vi "Write.vi"(0 "session in":T1[](array[typedef]) {"rx baseband session"."3630 session"."Address Space" items=["VXI/VME A16"=1, "VXI/VME A24"=2, "VXI/VME A32"=3, "VXI/VME A64"=4, "PXI Memory Allocations"=9, "PXI Configuration"=10, "PXI BAR0"=11, "PXI BAR1"=12, "PXI BAR2"=13, "PXI BAR3"=14, "PXI BAR4"=15, "PXI BAR5"=16]; "tx baseband session"."3610 session"."Address Space" items=["VXI/VME A16"=1, "VXI/VME A24"=2, "VXI/VME A32"=3, "VXI/VME A64"=4, "PXI Memory Allocations"=9, "PXI Configuration"=10, "PXI BAR0"=11, "PXI BAR1"=12, "PXI BAR2"=13, "PXI BAR3"=14, "PXI BAR4"=15, "PXI BAR5"=16]}, 1 "memo":enum16{"DRAM", "BRAM"}(ring), 5 "data":i16[](array[numeric]), 7 "Wfm addr":u32, 9 "zero pad":bool, 11 "error in":errorcluster) -> (3 "burst memo":enum16{"DRAM", "BRAM"}(ring), 4 "session out":T1[](array[typedef]) {"rx baseband session"."3630 session"."Address Space" items=["VXI/VME A16"=1, "VXI/VME A24"=2, "VXI/VME A32"=3, "VXI/VME A64"=4, "PXI Memory Allocations"=9, "PXI Configuration"=10, "PXI BAR0"=11, "PXI BAR1"=12, "PXI BAR2"=13, "PXI BAR3"=14, "PXI BAR4"=15, "PXI BAR5"=16]; "tx baseband session"."3610 session"."Address Space" items=["VXI/VME A16"=1, "VXI/VME A24"=2, "VXI/VME A32"=3, "VXI/VME A64"=4, "PXI Memory Allocations"=9, "PXI Configuration"=10, "PXI BAR0"=11, "PXI BAR1"=12, "PXI BAR2"=13, "PXI BAR3"=14, "PXI BAR4"=15, "PXI BAR5"=16]}, 6 "last wr addr":u32, 15 "error out":errorcluster)   [LabVIEW 2019, in "mmWave HW Control.lvlib"]
uses:
  mmWave HW Control.lvlib
  Low-level/TypeDefs/Session.ctl
  <instrlib>/niMmWave/ni3620/Config/v1/Host/Public/High-Level/niMmWave Session.ctl
  <instrlib>/_niInstr/Register Bus/v0/Host/Public/Register Bus Session.ctl
  <instrlib>/_niInstr/Register Bus/v0/Host/Private/Session Data.ctl
  <instrlib>/niMmWave/ni3620/Config/v1/Host/Public/Typedefs/Board Information.ctl
  <instrlib>/niMmWave/ni3620/Config/v1/Host/Public/Typedefs/Hardware Revision.ctl
  <instrlib>/niMmWave/ni3620/Config/v1/Host/Public/Typedefs/Gain Mapping.ctl
  <instrlib>/niMmWave/ni3620/Config/v1/Host/Public/Typedefs/Correction Data.ctl
  <instrlib>/niMmWave/ni3620/Config/v1/Host/Public/Typedefs/Opera Characterization.ctl
  <instrlib>/niMmWave/ni3620/Config/v1/Host/Public/Corrections/Typedefs/Opera Characterization Main Header.ctl
  <instrlib>/niMmWave/ni3620/Config/v1/Host/Public/Corrections/Typedefs/Opera IF Board Information.ctl
  <instrlib>/niMmWave/ni3620/Config/v1/Host/Public/Corrections/Typedefs/Opera Characterization Instance Header.ctl
  <instrlib>/niMmWave/ni3620/Config/v1/Host/Public/Corrections/Typedefs/Opera Characterization Device Data Header.ctl
  <instrlib>/niMmWave/ni3620/Config/v1/Host/Public/Corrections/Typedefs/Opera LO Characterization Data Header.ctl
  <instrlib>/niMmWave/ni3620/Config/v1/Host/Public/Corrections/Typedefs/Opera IF Board Characterization Data Header.ctl
  <instrlib>/niMmWave/ni3620/Config/v1/Host/Public/Corrections/Typedefs/Opera Characterization Device Data.ctl
  <instrlib>/niMmWave/ni3620/Config/v1/Host/Public/Corrections/Typedefs/Opera LO2 Board Characterization Data.ctl
  <instrlib>/niMmWave/ni3620/Config/v1/Host/Public/Corrections/Typedefs/Opera LO Characterization Data.ctl
  <instrlib>/niMmWave/ni3620/Config/v1/Host/Public/Corrections/Typedefs/Opera IF Board Characterization Data.ctl
  <instrlib>/niMmWave/ni3620/Config/v1/Host/Public/Corrections/Typedefs/Opera IQ Impairment Data.ctl
  <instrlib>/niMmWave/ni3620/Config/v1/Host/Public/Typedefs/mmWave Adapter Session Data.ctl
  <instrlib>/niMmWave/ni3620/Config/v1/Host/Public/Typedefs/mmWave Adapter Data.ctl
  <instrlib>/niMmWave/ni3620/Config/v1/Host/Public/Typedefs/mmWave Adapter 2.ctl
  <instrlib>/niMmWave/ni3620/Config/v1/Shared/Typedefs/Subsystem ID.ctl
  <instrlib>/niMmWave/ni3620/Config/v1/Host/Public/Typedefs/mmWave Adapter Channel Information.ctl
  <instrlib>/niMmWave/ni3620/Config/v1/Host/Public/Typedefs/Temperature Coefficients.ctl
  <instrlib>/niMmWave/ni3620/Config/v1/Host/Public/Typedefs/mmWave Characterization.ctl
  <instrlib>/niMmWave/ni3620/Config/v1/Host/Public/Corrections/Typedefs/mmWave Characterization Main Header.ctl
  <instrlib>/niMmWave/ni3620/Config/v1/Host/Public/Corrections/Typedefs/mmWave Characterization Instance Header.ctl
  <instrlib>/niMmWave/ni3620/Config/v1/Host/Public/Typedefs/Session Cache.ctl
  <instrlib>/niMmWave/ni3620/Config/v1/Host/Public/Typedefs/LO2 settings cache.ctl
  <instrlib>/niMmWave/ni3620/Config/v1/Host/Public/Typedefs/LO2 source.ctl
  <instrlib>/niMmWave/ni3620/Config/v1/Host/Public/Typedefs/Desired and Coerced.ctl
  <instrlib>/niMmWave/ni3620/Config/v1/Host/Public/Typedefs/Export cache.ctl
  <instrlib>/niMmWave/ni3620/Config/v1/Host/Public/Typedefs/Path cache.ctl
  <instrlib>/niMmWave/ni3620/Config/v1/Host/Public/Typedefs/Daughterboard Type.ctl
  <instrlib>/niMmWave/ni3620/Config/v1/Host/Public/Typedefs/LO1 settings cache.ctl
  <instrlib>/niMmWave/ni3620/Config/v1/Host/Public/Typedefs/LO1 Source.ctl
  <instrlib>/niMmWave/ni3620/Config/v1/Host/Public/Typedefs/mmWave export cache.ctl
  <instrlib>/niMmWave/ni3620/Config/v1/Host/Private/Board/LO2/LO2 Board Configuration Cache.ctl
  <instrlib>/niMmWave/ni3620/Config/v1/Host/Public/Typedefs/reference clock routing settings.ctl
  <instrlib>/niMmWave/ni3620/Config/v1/Host/Public/Typedefs/LO2 routing settings.ctl
  <instrlib>/niMmWave/ni3620/Config/v1/Host/Private/Board/LO1/LO1 Board Configuration Cache.ctl
  <instrlib>/niMmWave/ni3620/Config/v1/Host/Public/Typedefs/LO1 source settings.ctl
  <instrlib>/niMmWave/ni3620/Config/v1/Host/Public/Typedefs/LO1 export settings.ctl
  <instrlib>/niMmWave/ni3620/Config/v1/Host/Public/Typedefs/LO1 mmWave settings.ctl
  Low-level/TypeDefs/Tx Baseband Session.ctl
  <instrlib>/niMmWave/ni3610 and ni3630/controls/public/Main Settings.ctl
  <vilib>/Instr/_visa.llb/VISA Register Access Address Space.ctl
  <instrlib>/niMmWave/ni3610 and ni3630/controls/public/Register Adresses.ctl
  <instrlib>/niMmWave/ni3610 and ni3630/controls/public/Base Card Type.ctl
  <instrlib>/niMmWave/ni3610 and ni3630/controls/private/IQ Card Revision.ctl
  <instrlib>/niMmWave/ni3610 and ni3630/controls/public/Board Capability.ctl
  Low-level/TypeDefs/Blank FPGA Reference.ctl
  Low-level/TypeDefs/Rx Baseband Session.ctl
  Low-level/TypeDefs/Hardware Configuration.ctl
  Low-level/TypeDefs/Direction.ctl
  Low-level/TypeDefs/Gain Ranging.ctl
  Low-level/TypeDefs/PXI Trigger Bus Info.ctl
  Low-level/TypeDefs/TX driver FPGA ref.ctl
  00e56df4-ad1d-4d91-93ea-fba1cea4a9f5.vi
  38a8d631-9b78-4ee6-a370-a9c59af1ef2c.vi
  705eeaa0-497a-4033-9a85-e633e8683a5e.vi
  0942d1b7-6fcb-43fb-bb48-4a735e411df6.vi
  <vilib>/Utility/High Resolution Relative Seconds.vi
  <vilib>/Utility/error.llb/Clear Errors.vi
  <vilib>/rvi/errors/niLvFpgaAdjustHostInterfaceError.vi
  <vilib>/rvi/interface/common/niFpgaWaitOnOcc.vi
  <vilib>/rvi/interface/nirviReadWriteControl/nirviReadWriteControl.xnode
  <vilib>/rvi/interface/nirviMethod/nirviMethod.xnode
  NiFpgaLv.dll
  <vilib>/rvi/interface/Simulation/niFpgaSimulationCallBeginRW.vi
  <vilib>/rvi/errors/niLvFpgaMergeErrorWithErrorCode.vi
  <vilib>/FPGAPlugInAG/Dynamic/niLvFpga_ConfigureFifo_Dynamic.vi
  <vilib>/FPGAPlugInAG/Dynamic/niLvFpga_StartFifo_Dynamic.vi
  <vilib>/FPGAPlugInAG/Dynamic/niLvFpga_WriteFifo_Dynamic.vi
  <instrlib>/_niInstr/Register Bus/v0/Host/niInstr Register Bus v0 Host.lvlib
  <instrlib>/niMmWave/ni3610 and ni3630/ni3610_and_ni3630_Driver_Lib.lvlib
  <instrlib>/niMmWave/ni3620/Config/v1/Host/niMmWave Config v1 Host.lvlib
  <instrlib>/niMmWave/ni3620/Config/v1/Shared/niMmWave Config v1 Shared.lvlib
panel:
  out "conversion time":dbl format="%#_6p"
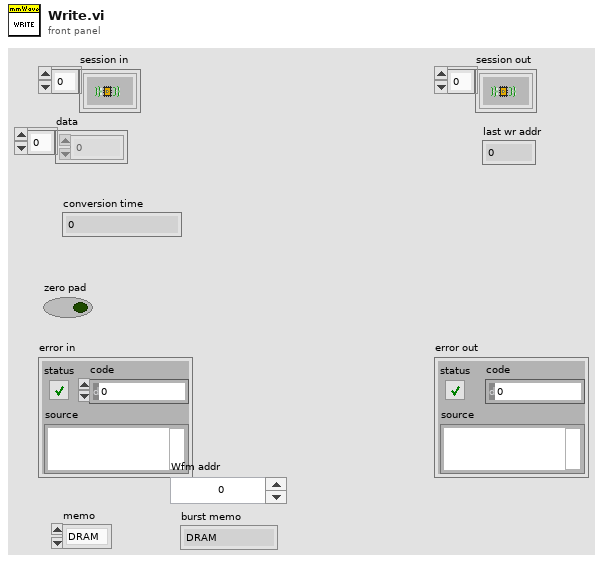
[diagram p1: front panel]
types:
  T1 = typedef "Session.ctl" = cluster{"3620 session":refnum<queue>, "tx baseband session":T2, "rx baseband session":T10, "tx gain (dB)":dbl, "rx gain (dB)":dbl, "hardware configuration":T11, "gain ranging":T13[], "pxi trigger bus information":T14}
  T2 = typedef "Tx Baseband Session.ctl" = cluster{"3610 session":T3, "7902 reference":T9}
  T3 = typedef "ni3610_and_ni3630_Driver_Lib.lvlib/Main Settings.ctl" = cluster{"VISA resource name":refnum<visa-resource-name>, "Address Space":T4, "window_offset":u32, "register_addresses":T5, "required_MM_fpga_version":cluster{"signature":u32, "hardware":u32, "current revision":u32, "oldest revision":u32}, "CPLD Oldest Compat Version ":cluster{"hardware":u32, "CPLD firmware":u32}, "MM_FPGA_image_location":string, "is_init":bool, "card_type":T6, "DacLmkConfigFileName":string, "AdcLmkConfigFileName":string, "AdcConfigFileName":string, "DacConfigFileName_RevA":string, "DacConfigFileName_RevB":string, "Mulde hardware revision":u8, "bypass DAC PLL\n":bool, "IQ Card Revision":T7, "board capability":T8}
  T4 = typedef "VISA Register Access Address Space.ctl" = u16
  T5 = typedef "ni3610_and_ni3630_Driver_Lib.lvlib/Register Adresses.ctl" = cluster{"MM based Registers":cluster{"Revision":u32, "OldestCompatRev":u32, "signature":u32, "scratch":u32, "LedControl":u32, "BoardHwRev":u32, "BoardControl":u32, "ThermalStatus":u32, "BasebandStatus":u32, "BasebandControl":u32, "BasebandAuxSetup":u32, "BasebandAuxStatus":u32, "LmkSyncOutSetup":u32, " AdcSyncOutSetup":u32, " InjSyncOutSetup":u32, " PxiTrig0OutSetup":u32, " PxiTrig1OutSetup":u32, " PxiTrig2OutSetup":u32, " PxiTrig3OutSetup":u32, " PxiTrig4OutSetup":u32, " PxiTrig5OutSetup":u32, " PxiTrig6OutSetup":u32, " PxiTrig7OutSetup":u32}, "CPLD based Registers":cluster{"SlaveSignature":u32, "SlaveRevision":u32, "SlaveOldestCompatRev":u32, "SlaveScratch":u32, "SlaveSetup":u32, "SlaveStatus":u32, "IDacReg_offset":u32, "LMKRegGrp0_offset":u32, "QDacReg_offset":u32, "BrdTempSensorVal":u32, "TempSensorPowerDown":u32, "GPIOReg_offset":u32, "IAdcReg_offset":u32, "QAdcReg_offset":u32, "LMKRegGrp1_offset":u32, "QadcTempSensorVal":u32, "IadcTempSensorVal":u32, "RevisionReg":u32, "VcxoReg":u32, "CpldStatusReg":u32, "PowerReg":u32, "VBiasEnReg":u32, "ExtRefOeReg":u32, "QdacCtrlReg":u32, "QdacStatusReg":u32, "IdacCtrlReg":u32, "IdacStatusReg":u32, "QdacJtagIn":u32, "QdacJtagOut":u32, "IdacJtagIn":u32, "IdacJtagOut":u32, "IqDcSetupReg":u32, "QadcStatusReg":u32, "IadcStatusReg":u32, "BrdSetupReg":u32, "IqDcRevisionReg":u32, "PllStatusReg":u32, "EndpointScratchReg":u32, "AdcSyncCfgReg":u32, "IqCardOpampReg":u32}, "CPLD Register Offset":u32, "MM  Register Offset":u32, " PxiTrig0OutSetup":u32}
  T6 = typedef "ni3610_and_ni3630_Driver_Lib.lvlib/Base Card Type.ctl" = enum16{"unspecified", "ADC", "DAC"}
  T7 = typedef "ni3610_and_ni3630_Driver_Lib.lvlib/IQ Card Revision.ctl" = enum16{"RevA", "RevB", "RevC", "RevD"}
  T8 = typedef "ni3610_and_ni3630_Driver_Lib.lvlib/Board Capability.ctl" = cluster{"baseband sync":enum16{"no baseband sync", "baseband sync"}}
  T9 = typedef "Blank FPGA Reference.ctl" = refnum<k20>
  T10 = typedef "Rx Baseband Session.ctl" = cluster{"3630 session":T3, "7902 reference":T9}
  T11 = typedef "Hardware Configuration.ctl" = cluster{"direction":T12, "baseband only":bool}
  T12 = typedef "Direction.ctl" = enum16{"Transceiver", "Receiver", "Transmitter"}
  T13 = typedef "Gain Ranging.ctl" = cluster{"gain ranging active scope":string, "gain ranging stream session":refnum<k20>}
  T14 = typedef "PXI Trigger Bus Info.ctl" = cluster{"chassis resource name":refnum<visa-resource-name>, "7902R (TX)":i16, "3610 (TX)":i16, "3620 (IF)":i16, "3630 (RX)":i16, "7902R (RX)":i16}
  T15 = cluster{"generation select":enum16{"Pass Through", "Tone", "Pulse", "Disable"}, "tone parameters":cluster{"frequency":fxp<+/-,48,0>, "gain":fxp<+/-,18,1>}, "pulse parameters":cluster{"frequency":u32, "gain":fxp<+/-,18,1>, "width":u8}}
  T16 = typedef "TX driver FPGA ref.ctl" = refnum<k20>
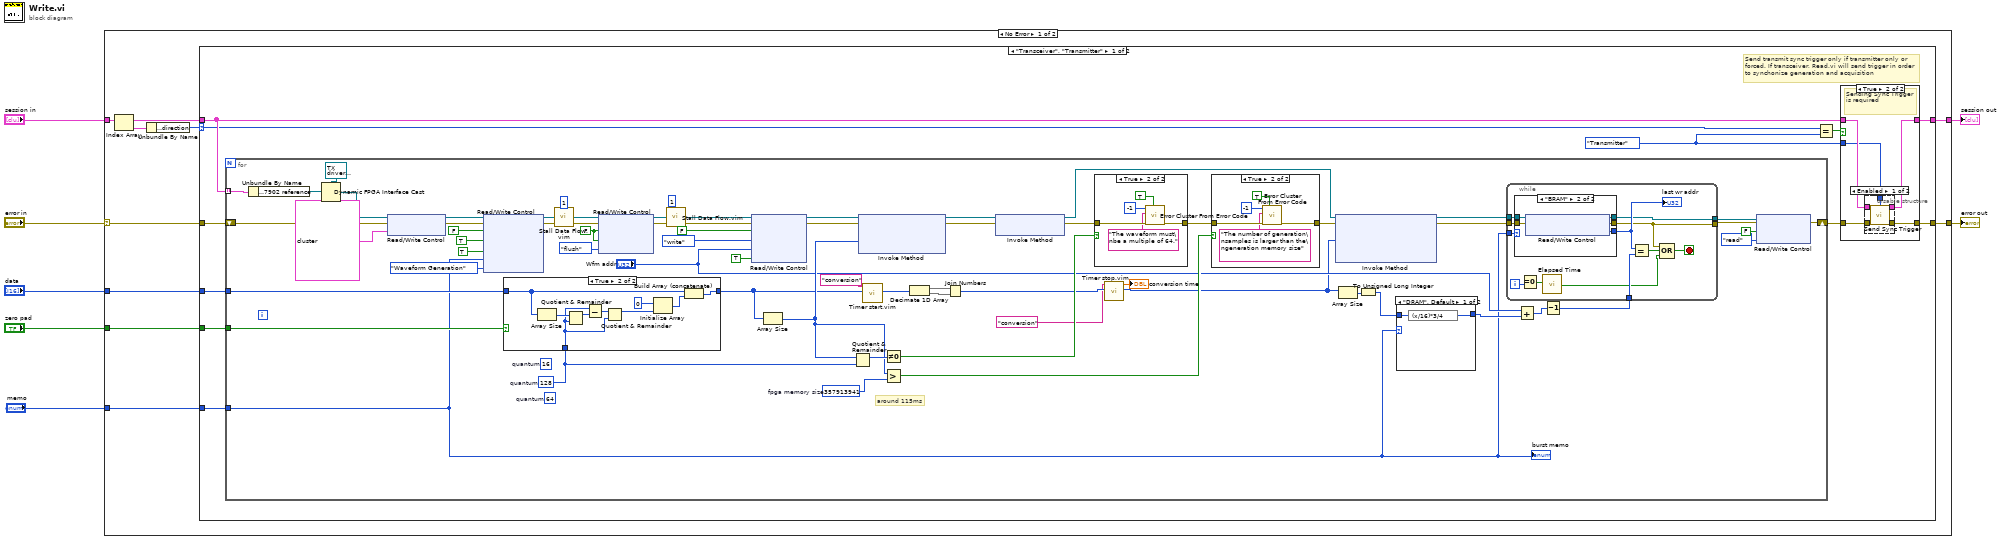
[diagram p0: block diagram]
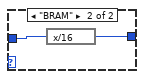
[diagram p4: hidden frame]
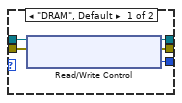
[diagram p5: hidden frame]
diagram:
  n1 = case shown="No Error" "error in" {
    selector: "error in" -> [w16 w157]
    tunnel: "session in" -> [w13 w156]
    tunnel: [w14 w157] -> w6
    tunnel: "zero pad" -> [w15 _]
    tunnel: [w10 w156] -> w3
    tunnel: "data" -> [w9 _]
    tunnel: "memo" -> [w8 _]
    frame No Error {
      n2 = Index Array(array=w13) -> (element=w12:T1)  [unwired: 1 in]
      n3 = Unbundle By Name(w12) -> ("hardware configuration.direction"=w11:T12)
      n4 = case shown="\"Transceiver\", \"Transmitter\"" w11 {
        selector: w11 -> [w21 _]
        tunnel: w16 -> [w27 w155]
        tunnel: w15 -> [w26 _]
        tunnel: [w24 w155] -> w14
        tunnel: w13 -> [w23 w154]
        tunnel: [w22 w154] -> w10
        tunnel: w9 -> [w18 _]
        tunnel: w8 -> [w17 _]
        frame "Transceiver", "Transmitter" {
          w20 = Direction."Transmitter" ("sync select")
          # "Send transmit sync trigger only if transmitter only or\nforced. If transceiver, Read.vi will send trigger in order\nto synchonize generation and acquisition"
          n5 = for {
            shift-right: [w69] -> w25
            shift-left: w27 -> [w45]
            tunnel: w23 -> [w95] mode=indexing
            tunnel: w26 -> [w93]
            tunnel: w18 -> [w91]
            tunnel: w17 -> [w57]
            (unwired) 64  # quantum
            w68 = u32 357913941  # fpga memory size
            w59 = FALSE
            w90 = 128  # quantum
            (unwired) 16  # quantum
            # "around 115ms"
            n6 = Unbundle By Name(w95) -> ("tx baseband session.7902 reference"=w94:T9)
            n7 = Dynamic FPGA Interface Cast(Session In=T16 refnum ("TX FPGA ref"), Type=w94) -> (Session Out=w47:T16)
            n8 = xnode "Read/Write Control"("FPGA VI Reference In"=w47, "error in"=w45, "cal.generation"=T15 {"generation select"=enum."Pass Through", "tone parameters"={"frequency"=0.0, "gain"=0.0}, "pulse parameters"={"frequency"=0, "gain"=0.0, "width"=0}}) -> ("FPGA VI Reference Out"=w43:T16, "error out"=w44:errorcluster)
            n9 = xnode "Read/Write Control"("FPGA VI Reference In"=w43, "error in"=w44, "seq.continous"=FALSE, "seq.rst"=TRUE ("sequence.cont"), "memo.reset"=TRUE, "burst memo"=w57, "waveform type"=enum16{"Tone", "Waveform Generation"}."Waveform Generation") -> ("FPGA VI Reference Out"=w85:T16, "error out"=w88:errorcluster)
            n10 = case shown="True" w93 {
              tunnel: w91 -> [w144 w149]
              tunnel: w90 -> [_ w147]
              tunnel: [w144 w148] -> w55
              frame False {
              }
              frame True {
                n11 = Array Size(array=w149) -> (size(s)=w153:i32)
                n12 = Quotient & Remainder(x=w153, y=w147) -> (x-y*floor(x/y)=w152:i32)  [unwired: 1 out]
                n13 = Subtract(x=w147, y=w152) -> (x-y=w146:i32)
                n14 = Quotient & Remainder(x=w146, y=w147) -> (x-y*floor(x/y)=w145:i32)  [unwired: 1 out]
                n15 = Initialize Array(i16 0 ("element"), w145) -> (w151:i16[])
                n16 = Build Array (concatenate)(w149, w151) -> (w148:i16[])
              }
            }
            n17 = call "Stall Data Flow.vim"("value in"=w85, "milliseconds to wait"=u32 1) -> ("value out"=w87:T16)  [unwired: 1 out]
            n18 = xnode "Read/Write Control"("FPGA VI Reference In"=w87, "error in"=w88, "memo.reset"=w59, "gen.enable"=w59, "memo mode"=enum16{"flush", "reset", "write", "read"}."flush" ("dram mode")) -> ("FPGA VI Reference Out"=w86:T16, "error out"=w89:errorcluster)
            n19 = call "Stall Data Flow.vim"("value in"=w86, "milliseconds to wait"=u32 1) -> ("value out"=w63:T16)  [unwired: 1 out]
            n20 = xnode "Read/Write Control"("FPGA VI Reference In"=w63, "error in"=w89, "iq.load"=FALSE, "memo mode"=enum16{"flush", "reset", "write", "read"}."write" ("dram mode"), "iq.load addr"="Wfm addr", "iq.load"=TRUE ("write/read")) -> ("FPGA VI Reference Out"=w78:T16, "error out"=w79:errorcluster)
            n21 = Array Size(array=w55) -> (size(s)=w102:i32)
            n22 = Quotient & Remainder(x=w102, y=w90) -> (x-y*floor(x/y)=w103:i32)  [unwired: 1 out]
            n23 = xnode "Invoke Method"("FPGA VI Reference In"=w78, "error in"=w79, "Requested Depth"=w102) -> ("FPGA VI Reference Out"=w105:T16, "error out"=w104:errorcluster)  [unwired: 1 out]
            n24 = call "Timer start.vim"("dataflow in"=w55, "timer name (t1)"="conversion") -> ("dataflow out"=w50:i16[])  [unwired: 9 in]
            n25 = Not Equal To 0?(x=w103) -> (x != 0?=w100:bool)
            n26 = Greater?(x=w102, y=w68) -> (0:w97:bool)
            n27 = Decimate 1D Array(w50) -> (w49:i16[], w48:i16[])
            n28 = Join Numbers(hi=w49, lo=w48) -> ((hi.lo)=w54:u32[])
            n29 = xnode "Invoke Method"("FPGA VI Reference In"=w105, "error in"=w104) -> ("FPGA VI Reference Out"=w99:T16, "error out"=w101:errorcluster)
            n30 = case shown="True" w100 {
              tunnel: w101 -> [w138 w143]
              tunnel: [w138 w142] -> w98
              frame False {
              }
              frame True {
                n31 = call <vilib>:"Error Cluster From Error Code.vi"("show call chain? (False)"=TRUE, "error in (no error)"=w143, "error message (\"\")"="The waveform must\nbe a multiple of 64." ("source"), "error code (0)"=-1) -> ("error out"=w142:errorcluster)  [unwired: 5 in]
              }
            }
            n32 = call "Timer stop.vim"("dataflow in"=w54, "timer name (t1)"="conversion") -> ("dataflow out"=w52:u32[], "final time"=→"conversion time":dbl)  [unwired: 8 in]
            n33 = case shown="True" w97 {
              tunnel: w98 -> [w132 w137]
              tunnel: [w132 w136] -> w96
              frame False {
              }
              frame True {
                n34 = call <vilib>:"Error Cluster From Error Code.vi"("show call chain? (False)"=TRUE, "error in (no error)"=w137, "error message (\"\")"="The number of generation\nsamples is larger than the\ngeneration memory size" ("source"), "error code (0)"=-1) -> ("error out"=w136:errorcluster)  [unwired: 5 in]
              }
            }
            n35 = xnode "Invoke Method"("FPGA VI Reference In"=w99, "error in"=w96, "Data"=w52) -> ("FPGA VI Reference Out"=w75:T16, "error out"=w74:errorcluster)  [unwired: 1 in, 1 out]
            n36 = Array Size(array=w52) -> (size(s)=w77:i32)
            n37 = To Unsigned Long Integer(number=w77) -> (unsigned 32bit integer=w66:u32)
            n38 = case shown="\"DRAM\", Default" w57 {
              tunnel: w66 -> [w107 w109]
              tunnel: [w106 w108] -> w65
              frame "DRAM", Default {
                n39 = expression code="(x/16)*3/4"(w107) -> (w106:u32)
              }
              frame "BRAM" {
                n40 = expression code="x/16"(w109) -> (w108:u32)
              }
            }
            n41 = Add(x="Wfm addr", y=w65) -> (x+y=w73:u32)
            n42 = Decrement(x=w73) -> (x-1=w67:u32)
            n43 = while {
              tunnel: w75 -> [w121]
              tunnel: w74 -> [w120]
              tunnel: w67 -> [w118]
              tunnel: [w115] -> w71
              tunnel: [w114] -> w70
              tunnel: w57 -> [w110]
              i -> [w112]
              stop <- w116 stop-if-true
              n44 = case shown="\"BRAM\"" w110 {
                tunnel: w121 -> [w126 w131]
                tunnel: w120 -> [w125 w130]
                tunnel: [w124 w129] -> w119
                tunnel: [w123 w128] -> w115
                tunnel: [w122 w127] -> w114
                frame "DRAM", Default {
                  n45 = xnode "Read/Write Control"("FPGA VI Reference In"=w126, "error in"=w125) -> ("FPGA VI Reference Out"=w122:T16, "error out"=w123:errorcluster, "dram.last written addr"=w124:u32)
                }
                frame "BRAM" {
                  n46 = xnode "Read/Write Control"("FPGA VI Reference In"=w131, "error in"=w130) -> ("FPGA VI Reference Out"=w127:T16, "error out"=w128:errorcluster, "bram.last written addr"=w129:u32)
                }
              }
              "last wr addr" <- w119
              n47 = Equal To 0?(x=w112) -> (x = 0?=w111:bool)
              n48 = call "Elapsed Time"("Reset"=w111) -> ("Time has Elapsed"=w113:bool)  [unwired: 11 in, 7 out]
              n49 = Equal?(x=w119, y=w118) -> (x = y?=w117:bool)
              n50 = Compound Arithmetic op=OR(w115, w117, w113) -> (w116:bool)
            }
            n51 = xnode "Read/Write Control"("FPGA VI Reference In"=w70, "error in"=w71, "iq.load"=FALSE, "memo mode"=enum16{"flush", "reset", "write", "read"}."read") -> ("error out"=w69:errorcluster)  [unwired: 1 out]
            "burst memo" <- w57
          }
          n52 = Equal?(x=w21, y=w20) -> (x = y?=w19:bool)
          n53 = case shown="True" w19 {
            tunnel: w25 -> [w28 w34]
            tunnel: [w28 w33] -> w24
            tunnel: w23 -> [w29 w32]
            tunnel: [w29 w31] -> w22
            tunnel: w20 -> [_ w30]
            frame False {
            }
            frame True {
              # "Sending Sync Trigger\nis required"
              n54 = disable-structure shown="Enabled" {
                disable-tunnel: w34 -> [w39 w40]
                disable-tunnel: [w38 w40] -> w33
                disable-tunnel: w32 -> [w37 w41]
                disable-tunnel: [w36 w41] -> w31
                disable-tunnel: w30 -> [w35 _]
                frame Enabled {
                  n55 = call "Send Sync Trigger.vi"("session in"=w37, "sync select"=w35, "error in"=w39) -> ("session out"=w36:T1[], "error out"=w38:errorcluster)  [unwired: 11 in]
                }
                frame Disabled {
                }
              }
            }
          }
        }
        frame "Receiver" {
        }
      }
    }
    frame Error {
    }
  }
  "session out" <- w3
  "error out" <- w6
